vi "Result_Test.vi"(8 "error in (no error)":errorcluster caption="entrée d'erreur (pas d'erreur)", 11 "Get_Voltage en entrée":refnum<class "Zigbee_Send_Msg_CH2.lvclass">) -> (0 "error out":errorcluster caption="sortie d'erreur", 3 "Get_Voltage en sortie":refnum<class "Zigbee_Send_Msg_CH2.lvclass">)   [LabVIEW 2020, in "Library Test.lvlib" / "Zigbee_Send_Msg_CH2.lvclass"]
uses:
  Zigbee_Send_Msg_CH2.lvclass
  C:/Users/ngarcin/OneDrive - Altyor/Standard TB/Suite TB45/Class/Test/Test (Default)/Test (Default).lvclass
  Commun VI/TypeDef/Variable Printable.ctl
  Zigbee_Send_Msg/Zigbee_Send_Msg.lvclass
  Commun VI/Library Commun.lvlib
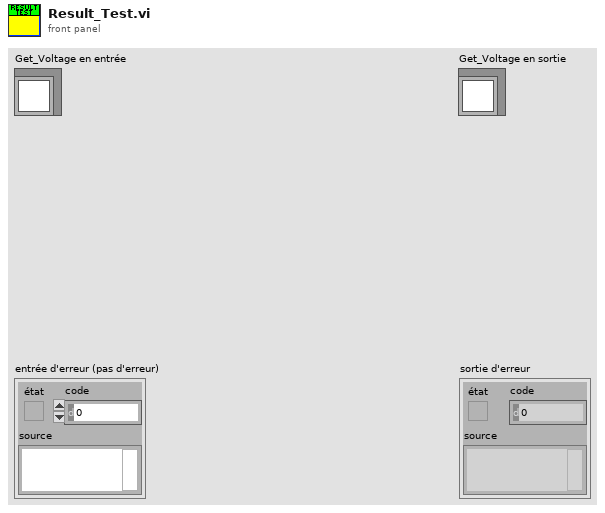
[diagram p1: front panel]
types:
  T1 = typedef "Variable Printable.ctl" = string
  T2 = enum16{"Get Variable", "Get All Variables", "Set Variable", "Delete Variable", "Delete All Variable"}
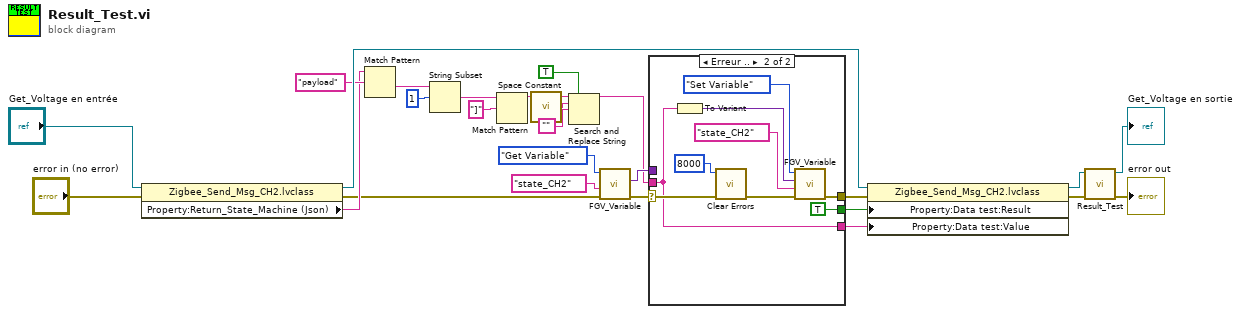
[diagram p0: block diagram]
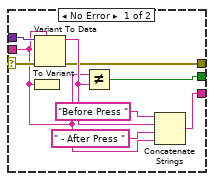
[diagram p2: hidden frame]
diagram:
  n1 = property class="Zigbee_Send_Msg_CH2.lvclass"(reference="Get_Voltage en entrée", error in="error in (no error)") -> (reference out=w26:refnum<class "Zigbee_Send_Msg_CH2.lvclass">, error out=w1:errorcluster, "Property:Return_State_Machine (Json)"=w10:string)
  n2 = Match Pattern(string=w10, regular expression="payload" ("expression régulière")) -> (after substring=w16:string)  [unwired: 1 in, 3 out]
  n3 = String Subset(string=w16, offset (0)=1) -> (substring=w15:string)  [unwired: 1 in]
  n4 = Match Pattern(string=w15, regular expression="]" ("expression régulière")) -> (before substring=w20:string)  [unwired: 1 in, 3 out]
  n5 = call <vilib>:"Space Constant.vi"() -> ("String"=w18:string)
  n6 = Search and Replace String(replace all?=TRUE ("tout remplacer ? (F)"), input string=w20, search string=w18, replace string="") -> (result string=w4:string)  [unwired: 4 in, 3 out]
  n7 = call "FGV_Variable.vi"("error in (no error)"=w1, "Variable"=T1 "state_CH2", "Function"=T2."Get Variable") -> ("error out"=w7:errorcluster, "Data Out"=w6:variant)  [unwired: 6 in, 1 out]
  n8 = case shown="Erreur .." w7 {
    selector: w7 -> [w35 w39]
    tunnel: [w27 w41] -> w3
    tunnel: w4 -> [w29 w36]
    tunnel: [w33 TRUE] -> w2
    tunnel: w6 -> [w34 _]
    tunnel: [w28 w36] -> w5
    frame No Error {
      n9 = To Variant(anything=w29) -> ()  [unwired: 1 out]
      n10 = Variant To Data(error in=w35, type=w29, Variant=w34) -> (data=w30:string, error out=w27:errorcluster)
      n11 = Not Equal?(x=w29, y=w30) -> (x != y?=w33:bool)
      n12 = Concatenate Strings("Before Press ", w30, " - After Press " ("chaîne"), w29) -> (w28:string)
    }
    frame Error {
      n13 = To Variant(anything=w36) -> (Variant=w42:variant)
      n14 = call <vilib>:"Clear Errors.vi"("error in (no error)"=w39, "specific error code to clear (0: all)"=8000) -> ("error out"=w37:errorcluster)  [unwired: 4 in, 1 out]
      n15 = call "FGV_Variable.vi"("error in (no error)"=w37, "Variable"=T1 "state_CH2", "Data In"=w42, "Function"=T2."Set Variable") -> ("error out"=w41:errorcluster)  [unwired: 5 in, 2 out]
    }
  }
  n16 = property class="Zigbee_Send_Msg_CH2.lvclass"(reference=w26, error in=w3, "Property:Data test:Result"=w2, "Property:Data test:Value"=w5) -> (reference out=w23:refnum<class "Zigbee_Send_Msg_CH2.lvclass">, error out=w25:errorcluster)
  n17 = call-parent "Result_Test.vi"("error in (no error)"=w25, "Get_Voltage en entrée"=w23) -> ("error out"=→"error out":errorcluster, "Get_Voltage en sortie"=→"Get_Voltage en sortie":refnum<class "Zigbee_Send_Msg_CH2.lvclass">)  [unwired: 8 in]
